vi "Define Correlator Port+.vi"(1 "VISA resource name":refnum<visa-resource-name>="COM1", 2 "Addr (0-15)":i8 min=0 max=15 step=1) -> ()   [LabVIEW 2012]
uses:
  Correlator port.vi
panel:
  in  "Define":bool
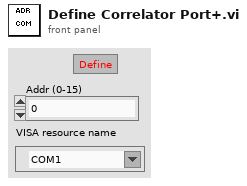
[diagram p1: front panel]
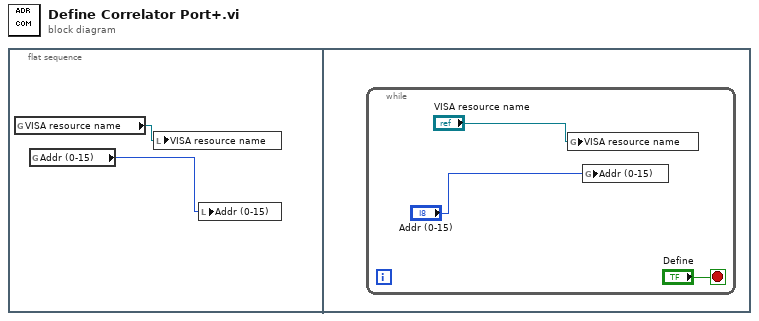
[diagram p0: block diagram]
diagram:
  n1 = flat-sequence {
    frame #0 {
      n2 = global read "Correlator port.vi" "VISA resource name"() -> (w1:refnum<visa-resource-name>)
      n3 = global read "Correlator port.vi" "Addr (0-15)"() -> (w2:i8)
      n4 = local write "VISA resource name"(w1) -> ()
      n5 = local write "Addr (0-15)"(w2) -> ()
    }
    frame #1 {
      n6 = while {
        stop <- "Define" stop-if-true
        n7 = global write "Correlator port.vi" "VISA resource name"("VISA resource name") -> ()
        n8 = global write "Correlator port.vi" "Addr (0-15)"("Addr (0-15)") -> ()
      }
    }
  }
